vi "UI.vi"(0 "reference in":refnum<class "GUI NV.lvclass">, 5 "error in (no error)":errorcluster) -> (14 "reference out":refnum<class "GUI NV.lvclass">, 19 "error out":errorcluster)   [LabVIEW 2019, in "GUI NV.lvclass"]
uses:
  GUI NV.lvclass
  C:/Users/ANENKOV_V1/Desktop/src/GUI_class/GUI.lvclass
  modbus engine custom/MB_ENGINE_class/Engine Alarms.ctl
  modbus engine custom/MB_ENGINE_class/Settings.ctl
  modbus engine custom/MB_ENGINE_class/cmd enum.ctl
  modbus engine custom/MB_ENGINE_class/Engine State.ctl
  TypeDef/Needle Valve Settings.ctl
  modbus engine custom/MB_ENGINE_class/Limits Status.ctl
  GUI_class/GUI.lvclass/GUI.ctl
  TypeDef/Needle Valve Data.ctl
  TypeDef/Needle Valve State.ctl
  SV_Wrap/SharedVariableWrapper.lvclass/SharedVariableWrapper.ctl
  MessageAMC_class/MessageAMC.lvclass
  C:/Users/ANENKOV_V1/Desktop/src/MessageInterface_class/MessageInterface.lvclass
  1d603503-2144-48e8-a995-f81b8b527575.vi
  8a81be2e-f949-43bf-aca8-28cc7a7f0a37.vi
  d3712f08-a2f0-4b08-adfd-5b0c4b698223.vi
  1b4fed76-272f-4eb9-b435-1b7916789d73.vi
  d0ca9bf2-7cd9-4c29-a03d-de1c10393a74.vi
  0872259c-c1b7-4622-8eff-96544e628326.vi
  9c882fec-a0e6-4663-a7fe-14c8a64433d0.vi
  GUI_class/Set Win State.vi
  GUI_class/protected/GetSheredData.vi
  1b4fed76-272f-4eb9-b435-1b7916789d73.vi/a620cbe0-d7b3-4cdc-ae28-4bc688216dd7.vi
  SV_Wrap/Write Var Info.vi
  SV_Wrap/Read Var Info.vi
  d0ca9bf2-7cd9-4c29-a03d-de1c10393a74.vi/168a1798-03ba-412e-8d8f-3bc5fd34782a.vi
  0872259c-c1b7-4622-8eff-96544e628326.vi/c08680f8-4eaf-4e08-9f5a-be355d832679.vi
  SV_Wrap/Read connection str.vi
  <userlib>/_OpenG.lib/time/time.llb/Tick Count (ms)__ogtk.vi
  GUI_class/GUI.lvclass
  MessageInterface_class/MessageInterface.lvclass
  SV_Wrap/SharedVariableWrapper.lvclass
  modbus engine custom/MB_ENGINE_class/MB_ENGINE.lvclass
panel:
  in  "stop 2":bool
  in  "clear chart":bool
  in  "ziro angl":bool
  out "Limits":T1
  out "Name":string
  in  "Needle Valve Settings":T2={"average size"=0, "open force"=12, "close force"=12, "open settings"={"ACC Steps Per Sec^2"=0, "DEC Steps Per Sec^2"=0, "Min Velosity Step Per Sec"=0, "Max Velosity Step Per Sec"=0, "MicroStep"=0}, "close settings"={"ACC Steps Per Sec^2"=0, "DEC Steps Per Sec^2"=0, "Min Velosity Step Per Sec"=0, "Max Velosity Step Per Sec"=0, "MicroStep"=0}, "Offset angle"=0.0} caption="Settings" {"close force" min=10 max=100; "open force" min=10 max=100; "average size" min=5 max=1000}
  in  "Engine State":T4 items=["ACCELERATING", "DECELERATINGTOSTOP", "DECELERATING", "STEADY", "INDEX_ACCEL", "NDEX_RUN", "INDEX_DECEL", "INDEX_DWELL", "INACTIVE", "STANDBY", "STANDBYTOINACTIVE"]
  out "String 2":string
  out "String":string
  in  "clear fault":bool
  in  "stop":bool
  in  "close":bool
  in  "open":bool
  in  "Set_cmd":bool
  in  "cmd to write":T5 items=["0 Idle"=0, "1 GoTo Absolute Position"=1, "2 GoTo Relative"=2, "10 GoTo Home Position"=10, "11 Set Home Position"=11, "12 Set FindHome Mode"=12, "13 Reset FindHome Mode"=13, "14 Get FindHome State"=14, "20 Hard Stop"=20, "21 HiZ Stop"=21, "22 Soft Stop"=22, "30 Clear Fault"=30, "40 Encoder Set Home"=40, "70 Driver Init"=70]
  out "Kinematic":T3
  out "Waveform Chart - Dark 3":dbl(graph) caption="Угол"
  out "encoder":i32(graph) caption="Энкодер"
  out "step":i32(graph) caption="ШАГ"
  out "Alarms":T6
  out "DO 19":bool
  out "Not Connect":bool caption="Подключение"
  in  "stop":bool
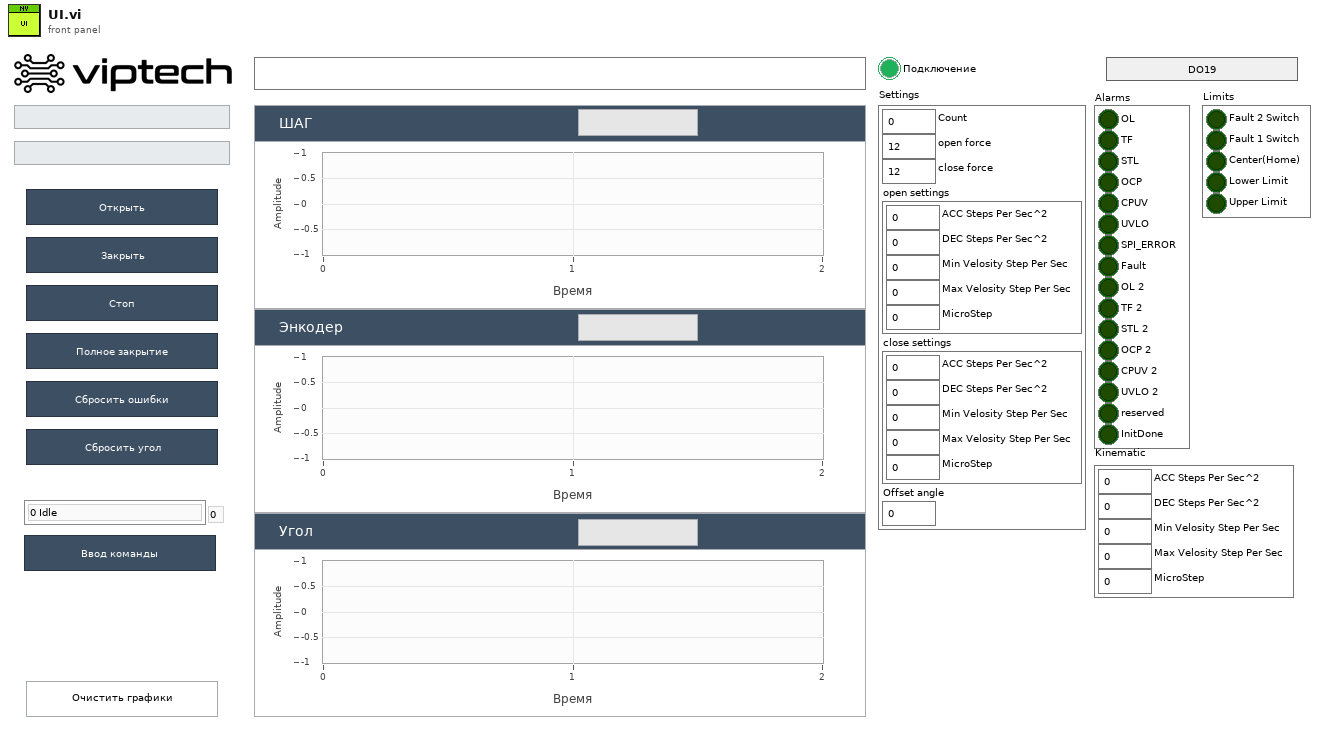
[diagram p1: front panel]
types:
  T1 = typedef "MB_ENGINE.lvclass/Limits Status.ctl" = cluster{"Fault 2 Switch":bool, "Fault 1 Switch":bool, "Center(Home)":bool, "Lower Limit":bool, "Upper Limit":bool}
  T2 = typedef "Needle Valve Settings.ctl" = cluster{"average size":i32, "open force":u16, "close force":u16, "open settings":T3, "close settings":T3, "Offset angle":dbl}
  T3 = typedef "MB_ENGINE.lvclass/Settings.ctl" = cluster{"ACC Steps Per Sec^2":u16, "DEC Steps Per Sec^2":u16, "Min Velosity Step Per Sec":u16, "Max Velosity Step Per Sec":u16, "MicroStep":u16}
  T4 = typedef "MB_ENGINE.lvclass/Engine State.ctl" = u16
  T5 = typedef "MB_ENGINE.lvclass/cmd enum.ctl" = u16
  T6 = typedef "MB_ENGINE.lvclass/Engine Alarms.ctl" = cluster{"OL":bool, "TF":bool, "STL":bool, "OCP":bool, "CPUV":bool, "UVLO":bool, "SPI_ERROR":bool, "Fault":bool, "OL 2":bool, "TF 2":bool, "STL 2":bool, "OCP 2":bool, "CPUV 2":bool, "UVLO 2":bool, "reserved":bool, "InitDone":bool}
  T7 = enum32{"Invalid", "Standard", "Closed", "Hidden", "Minimized", "Maximized"}
  T8 = enum32{"invalid app kind", "Development System", "Run Time System", "Student Edition", "Embedded LabVIEW", "Evaluation", "Custom"}
  T9 = typedef "SharedVariableWrapper.lvclass/Config.ctl" = cluster{"connection str":string, "timeout":dbl, "ip":string}
  T10 = cluster{"Core":cluster{"Current VI Reference":refnum<vi>, "Close Panel on Exit?":bool}, "amc":refnum<class "MessageAMC.lvclass">}
  T11 = cluster{"Current VI Reference":refnum<vi>, "Close Panel on Exit?":bool}
  T12 = typedef "Needle Valve Data.ctl" = cluster{"Engine State":T4, "StateValveModbus":T13, "Alarms":T6, "RAW":i32, "Angele":dbl, "Step":i32, "Encoder":i32, "Kinematic":T3, "Limits":T1, "EncoderMax":i32, "Counter Max Dont Update":i32, "EncoderMin":i32, "Counter Min Dont Update":i32, "Prepere Counter":i32, "STEP INIT":i32, "offset - Angel":dbl}
  T13 = typedef "Needle Valve State.ctl" = enum16{"STOPED", "CLOSED", "OPENED", "OPENING", "CLOSING", "FULL_CLOSE"}
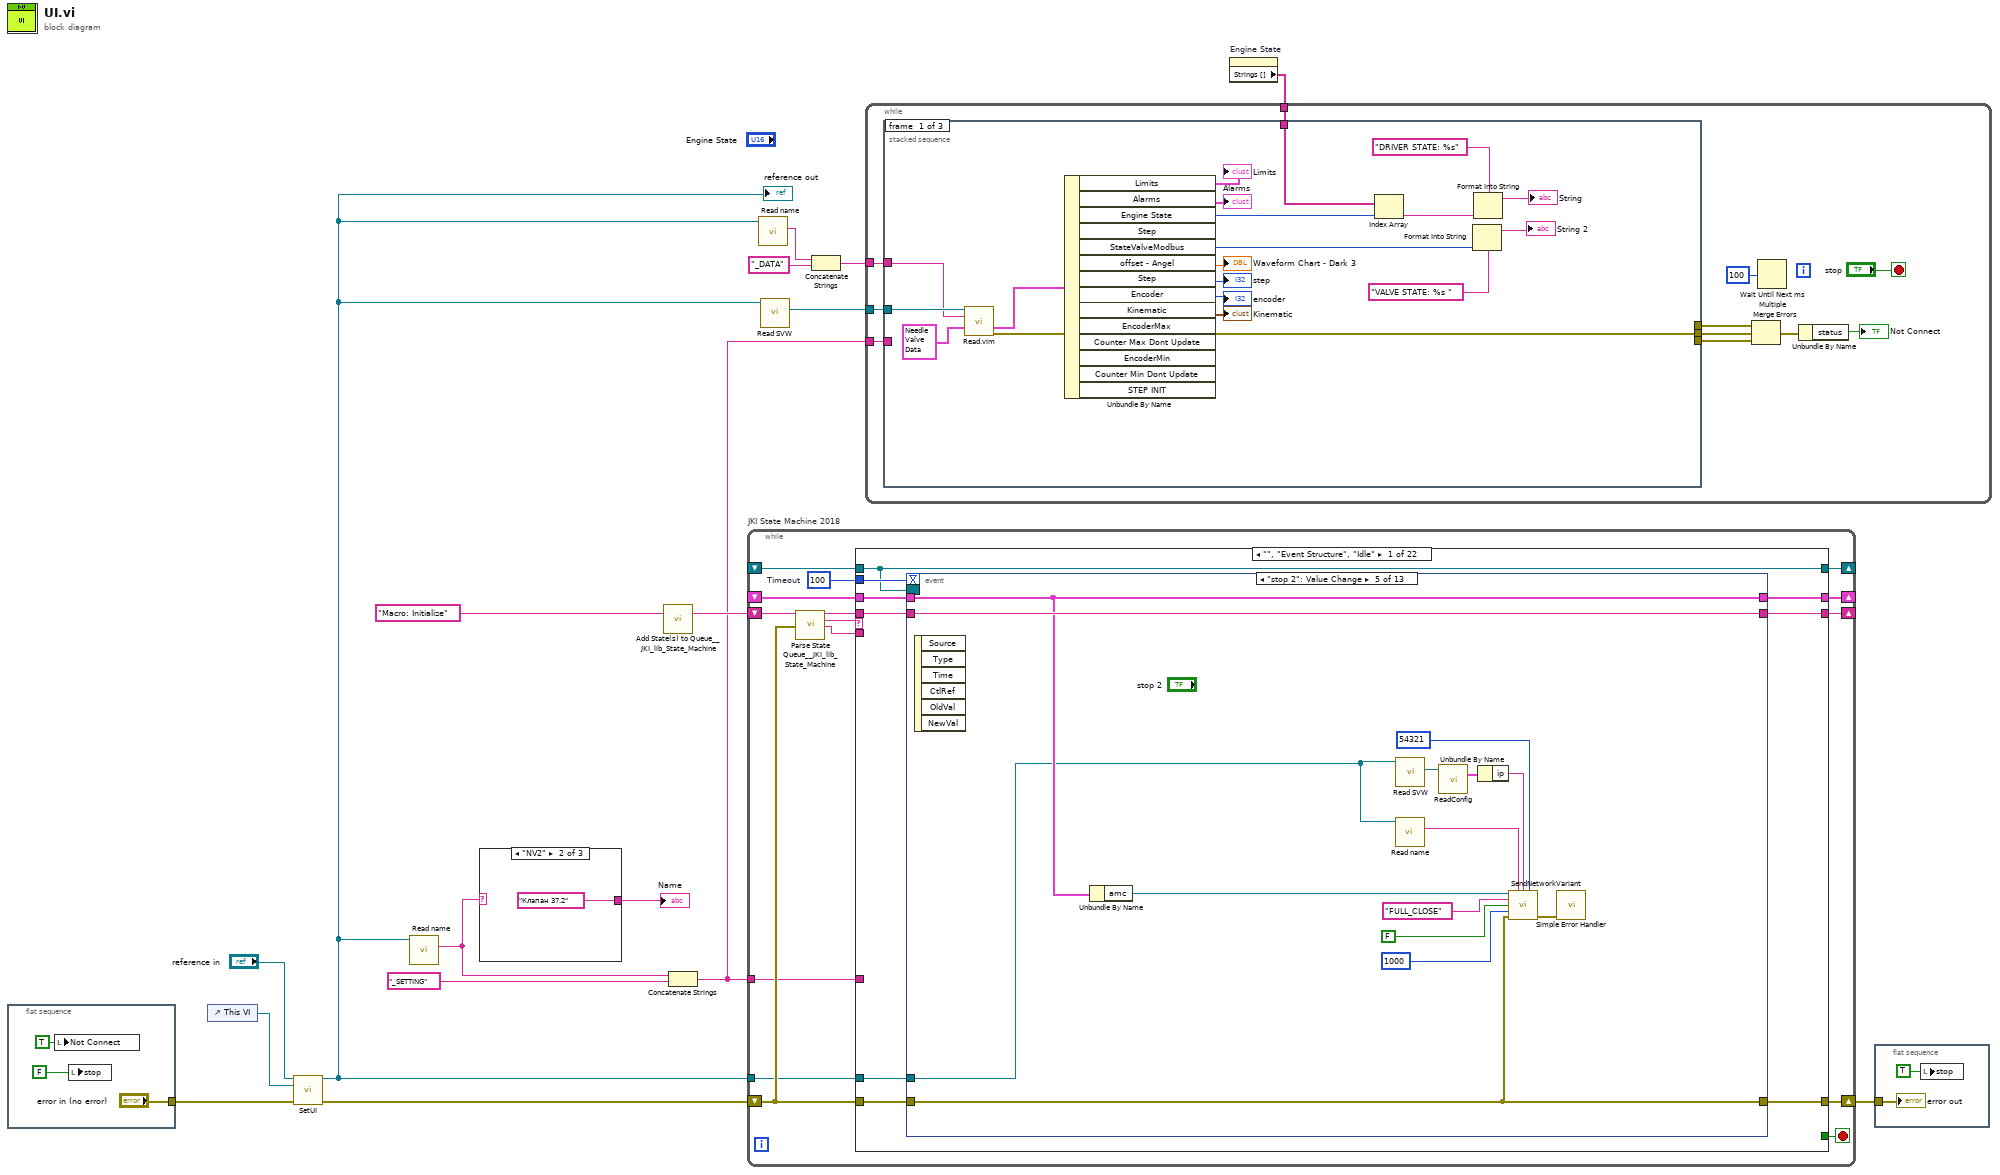
[diagram p0: block diagram]
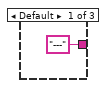
[diagram p2: hidden frame]
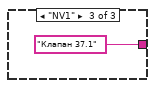
[diagram p3: hidden frame]
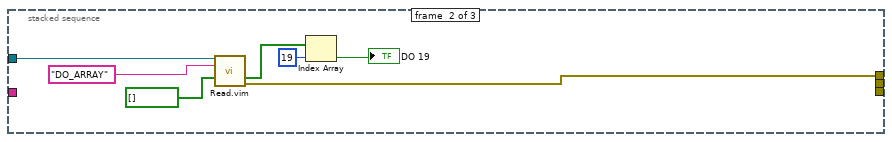
[diagram p4: hidden frame]
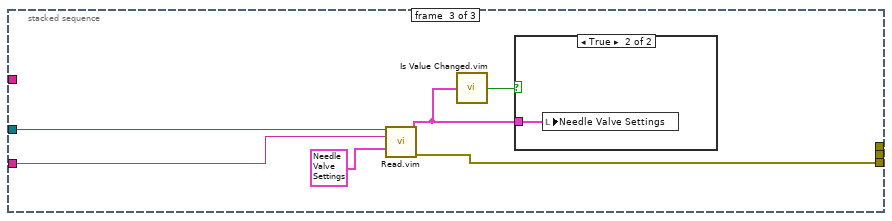
[diagram p5: hidden frame]
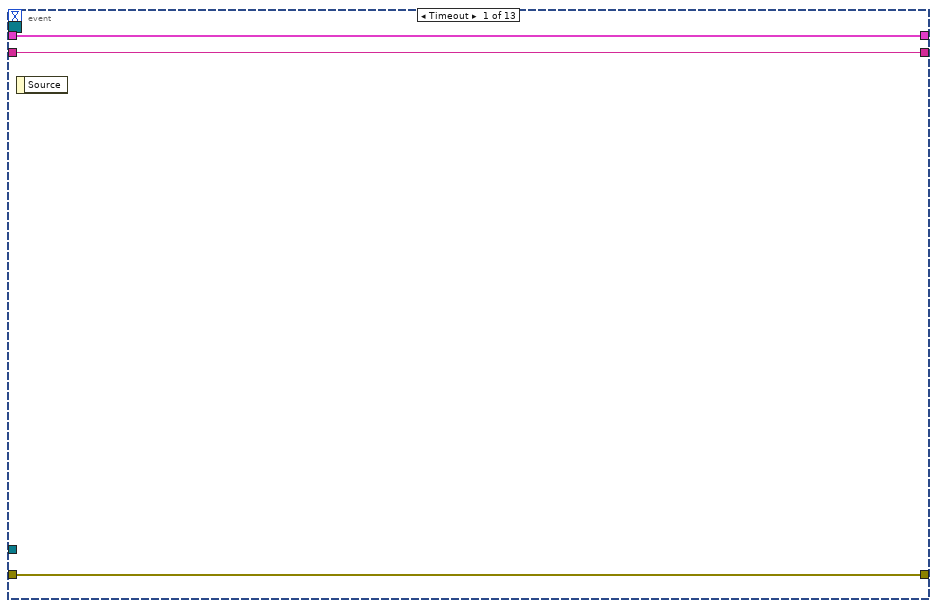
[diagram p7: hidden frame]
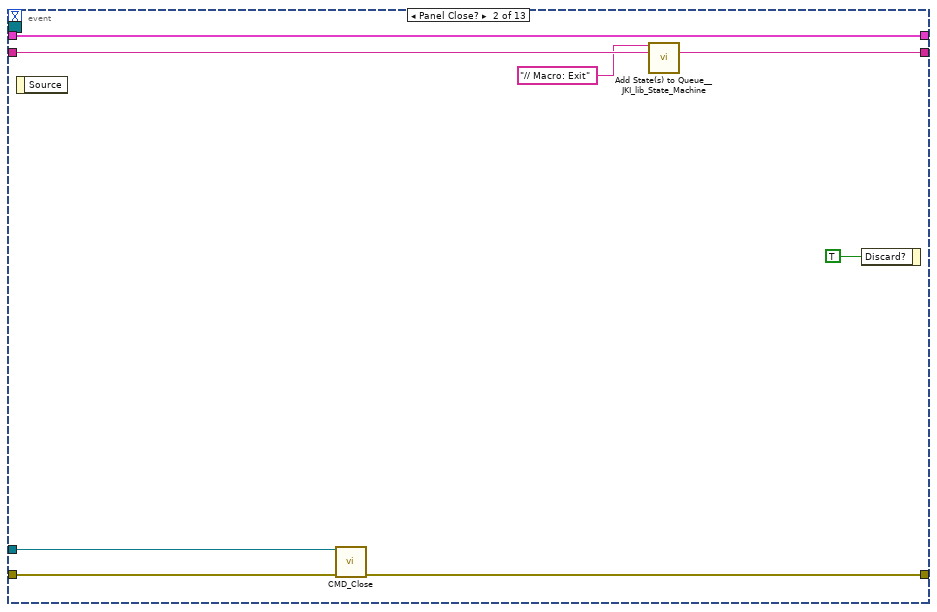
[diagram p8: hidden frame]
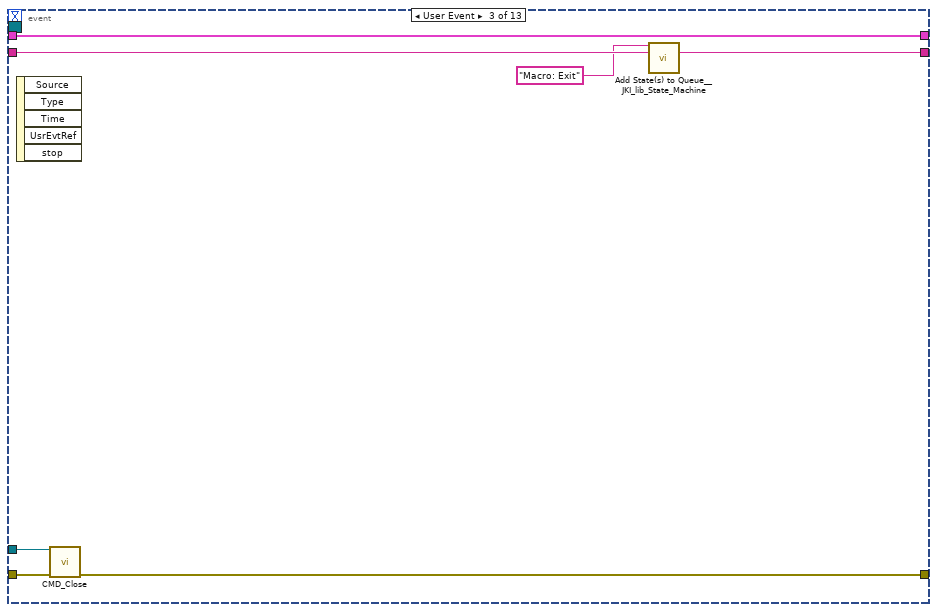
[diagram p9: hidden frame]
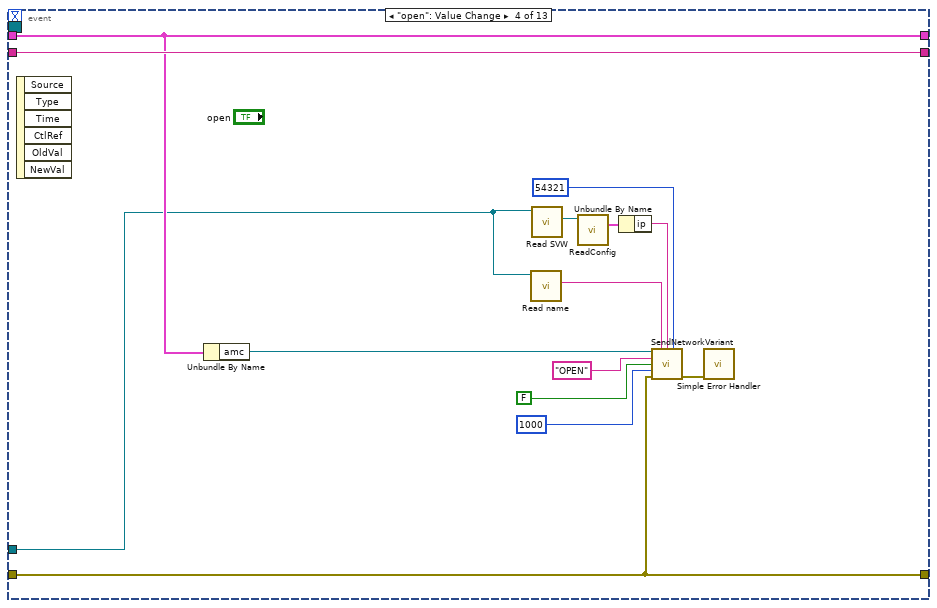
[diagram p10: hidden frame]
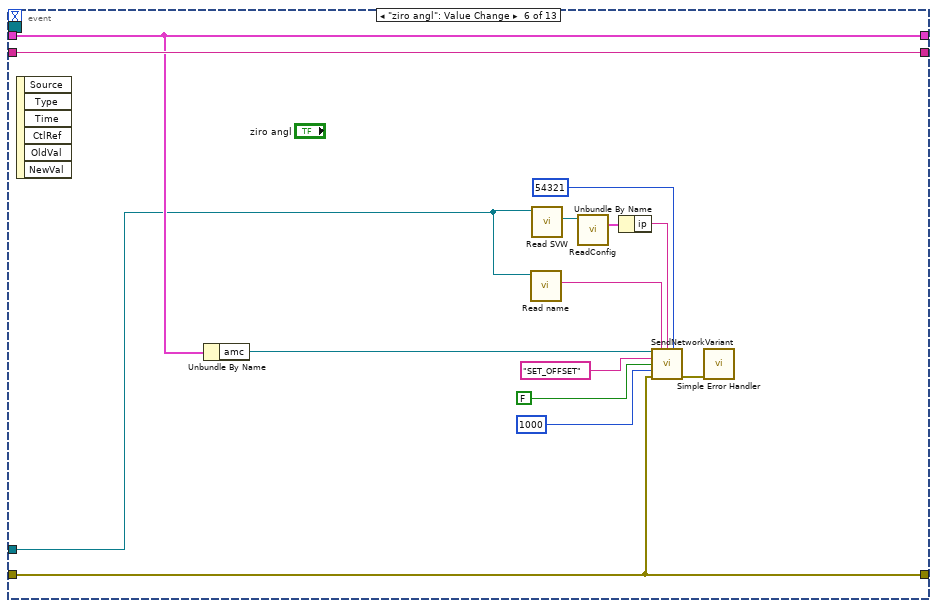
[diagram p11: hidden frame]
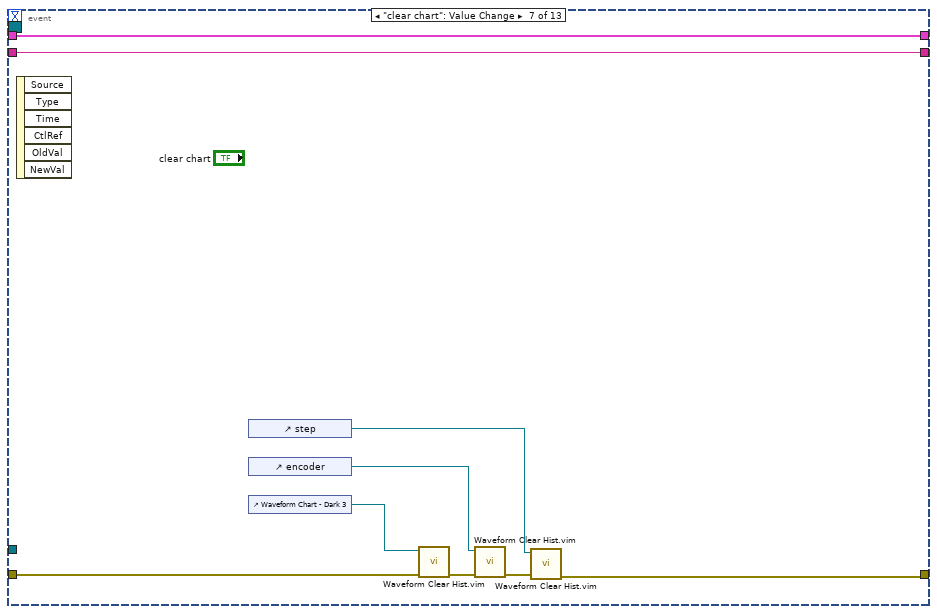
[diagram p12: hidden frame]
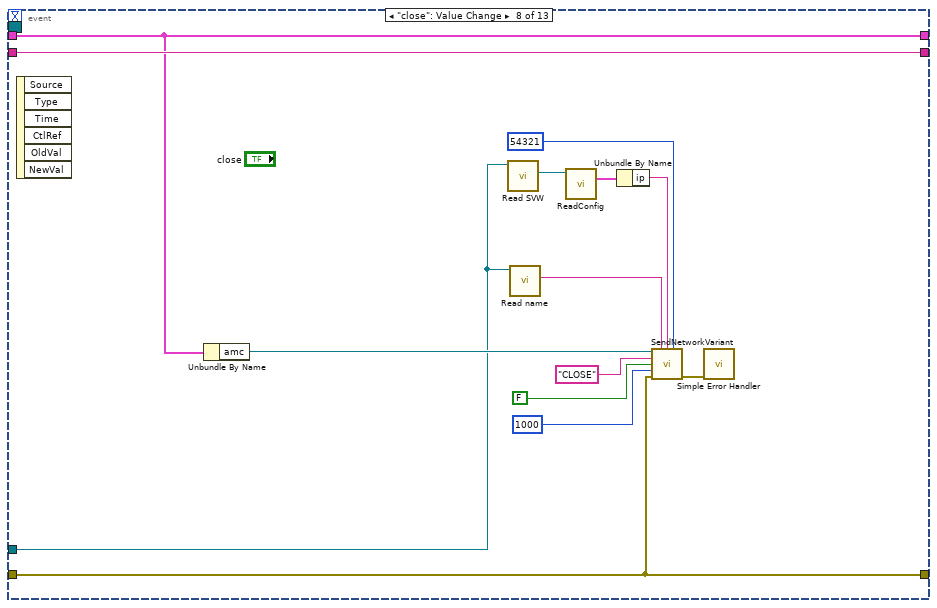
[diagram p13: hidden frame]
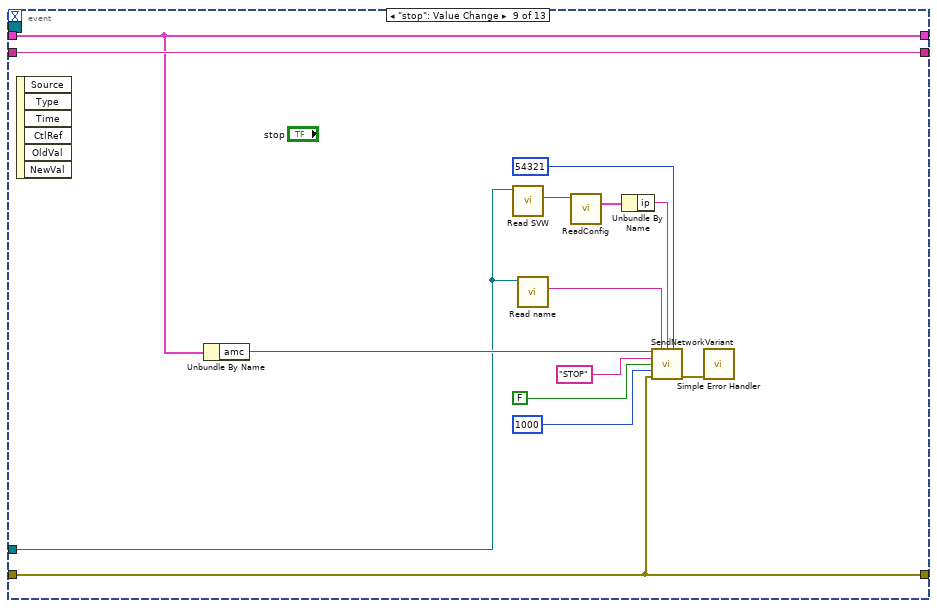
[diagram p14: hidden frame]
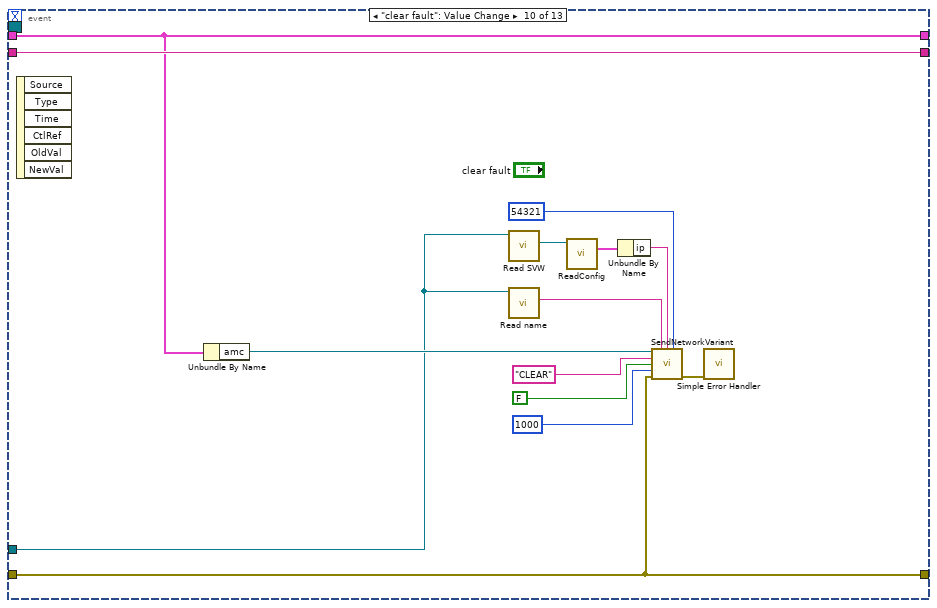
[diagram p15: hidden frame]
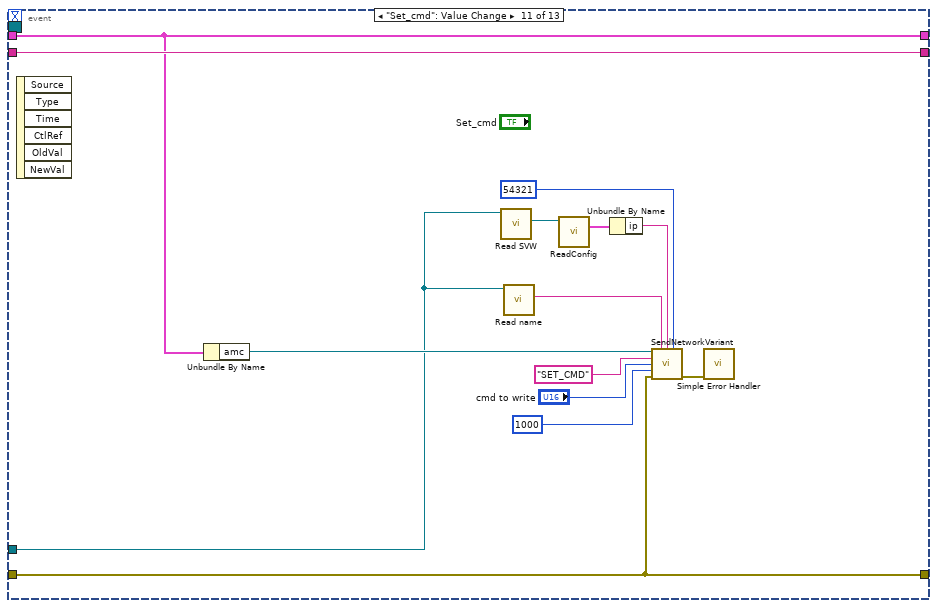
[diagram p16: hidden frame]
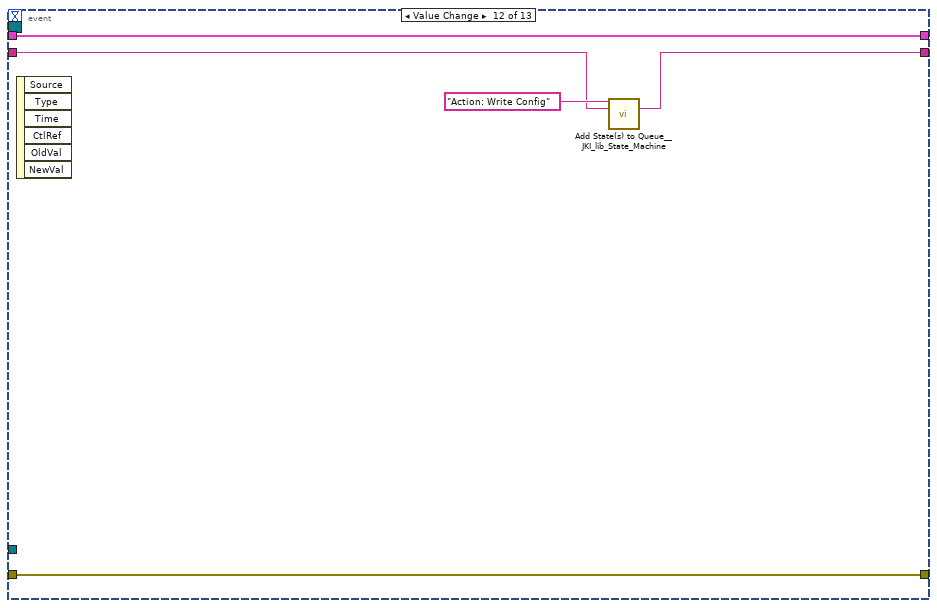
[diagram p17: hidden frame]
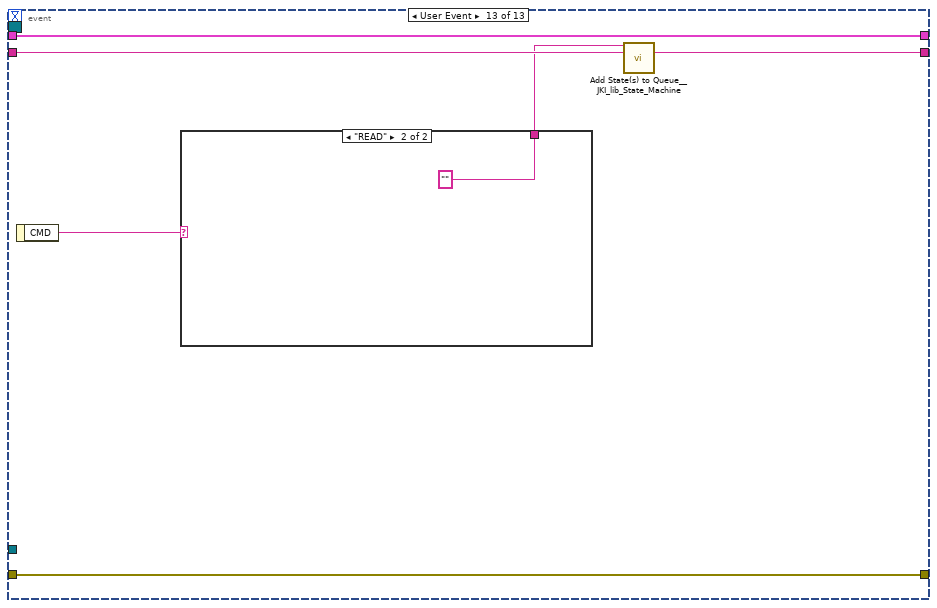
[diagram p18: hidden frame]
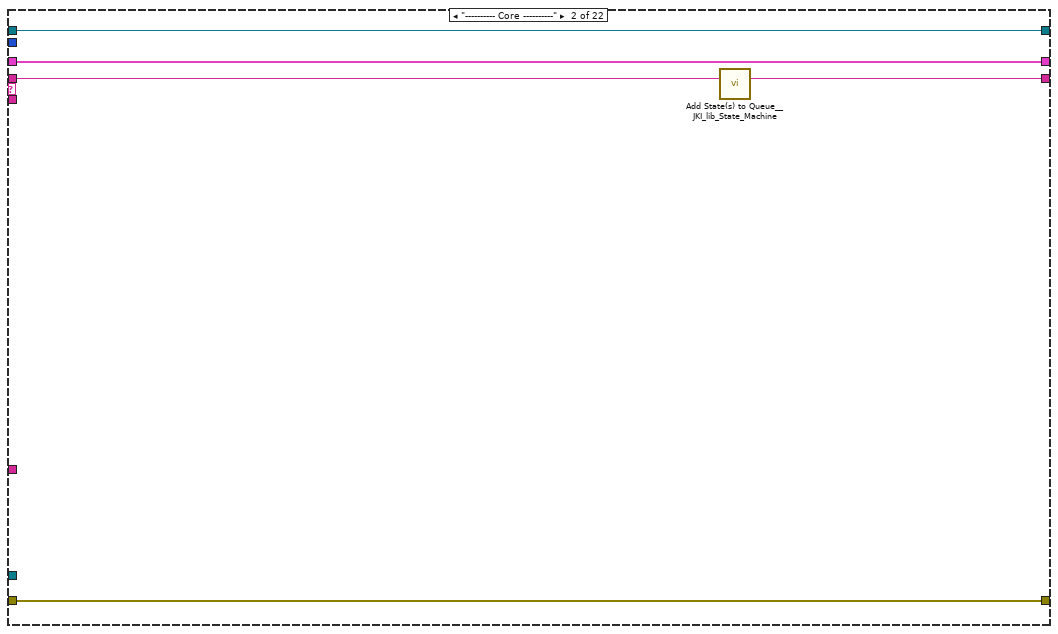
[diagram p20: hidden frame]
diagram:
  n1 = flat-sequence {
    tunnel: ["error in (no error)"] -> w14
    frame #0 {
      n2 = local write "Not Connect"(TRUE ("Connect")) -> ()
      n3 = local write "stop"(FALSE ("stop")) -> ()
    }
  }
  n4 = control-ref of="This VI"() -> (w12:refnum<vi>)
  n5 = call "SetUI.vi"("reference in"="reference in", "UI VI"=w12, "error in (no error)"=w14) -> ("reference out"=w4:refnum<class "GUI NV.lvclass">, "error out"=w11:errorcluster)  [unwired: 11 in]
  "reference out" <- w4
  n6 = call "Read name.vi"("GUI in"=w4) -> ("name"=w2:string)  [unwired: 9 in, 1 out]
  n7 = case shown="\"NV2\"" w2 {
    tunnel: ["---" "Клапан 37.2" "Клапан 37.1"] -> w1
    frame Default {
    }
    frame "NV2" {
    }
    frame "NV1" {
    }
  }
  "Name" <- w1
  n8 = call <vilib>:"Add State(s) to Queue__JKI_lib_State_Machine.vi"("State(s) in (\"\")"="Macro: Initialize") -> ("States Out"=w17:string)  [unwired: 14 in]
  n9 = Concatenate Strings(w2, "_SETTING" ("name")) -> (w3:string)
  n10 = while "JKI State Machine 2018" {
    shift-right: [w31] -> _
    shift-left: _ -> [w30]
    shift-right: [w34] -> w15
    shift-left: w11 -> [w28]
    shift-right: [w33] -> _
    shift-left: w17 -> [w35]
    tunnel: w4 -> [w27]
    shift-right: [w26] -> _
    shift-left: _ -> [w25]
    tunnel: w3 -> [w24]
    stop <- w32 stop-if-true
    w29 = 100  # Timeout
    n11 = call <vilib>:"Parse State Queue__JKI_lib_State_Machine.vi"("State Queue"=w35, "Error In (no error)"=w28) -> ("Remaining States"=w37:string, "Current State"=w38:string, "Arguments"=w36:string)  [unwired: 11 in]
    n12 = case shown="\"\", \"Event Structure\", \"Idle\"" w38 {
      selector: w38 -> [_ _ w191 _ _ _ _ _ _ _ _ _ _ _ _ _ _ _ _ _ _ _]
      tunnel: w37 -> [w47 w189 w195 w215 w222 w230 w235 w244 w251 w256 w264 w270 w275 w279 w286 w298 w368 w374 w380 w392 w396 w403]
      tunnel: w36 -> [_ _ _ _ _ _ _ _ _ _ _ _ _ _ w281 w292 _ _ _ _ _ _]
      tunnel: w30 -> [w45 w186 w193 w208 w219 w225 w232 _ w246 w253 w263 w268 w272 w278 w284 w294 w365 w371 w377 w389 w394 w398]
      tunnel: [w44 w187 w197 w212 errorcluster {"status"=FALSE, "code"=0, "source"=""} ("error out") w228 w233 w237 w247 w254 w261 w265 w273 w277 w282 w295 w366 w372 w378 w390 w395 w400] -> w34
      tunnel: w28 -> [w43 w187 w196 w212 w218 w228 w233 w238 w248 w254 w260 w266 w273 w277 w283 w296 w366 w372 w378 w390 w395 w401]
      tunnel: [w46 w188 w194 w214 w221 w229 w234 w244 w250 w255 w264 w269 w274 w279 w285 w297 w367 w373 w379 w391 w396 w403] -> w33
      tunnel: [_ _ _ _ _ TRUE _ _ _ _ _ _ _ _ _ _ _ _ _ _ _ _] -> w32
      tunnel: [w42 w186 w193 w213 w219 w225 w232 w243 w246 w253 w263 w268 w272 w278 w284 w294 w365 w371 w377 w389 w394 w398] -> w31
      tunnel: w29 -> [w41 _ _ _ _ _ _ _ _ _ _ _ _ _ _ _ _ _ _ _ _ _]
      tunnel: w27 -> [w40 _ _ _ _ _ _ _ _ _ w259 _ _ _ _ _ _ _ _ _ _ w399]
      tunnel: [w39 w185 w190 w202 w216 w226 w231 w241 w245 w252 w262 w267 w271 w276 w280 w291 w364 w369 w375 w382 w393 w402] -> w26
      tunnel: w25 -> [w39 w185 w190 w202 w216 w226 w231 w241 w245 w252 _ w267 w271 w276 w280 w291 w364 w369 w375 w382 w393 w402]
      tunnel: w24 -> [_ _ _ _ _ _ _ _ _ _ _ _ _ _ _ _ _ _ _ _ _ _]
      frame "", "Event Structure", "Idle" {
        n13 = event shown="[4] \"stop 2\": Value Change" {
          selector: w39 -> [_ _ _ _ _ _ _ _ _ _ _ _ _]
          dyn-events: _ -> [_ _ _ _ _ _ _ _ _ _ _ _ _]
          timeout: w41 -> [_ _ _ _ _ _ _ _ _ _ _ _ _]
          tunnel: w47 -> [w50 w58 w65 w79 w93 w107 w116 w130 w144 w158 w172 w174 w180]
          tunnel: [w50 w57 w64 w79 w93 w107 w116 w130 w144 w158 w172 w173 w181] -> w46
          tunnel: w45 -> [w48 w56 w63 w73 w87 w101 w115 w124 w138 w152 w166 w176 w182]
          tunnel: [w49 w51 w59 w68 w82 w96 w111 w119 w133 w147 w162 w177 w183] -> w44
          tunnel: w43 -> [w49 w52 w60 w68 w82 w96 w114 w119 w133 w147 w162 w177 w183]
          tunnel: [w48 w56 w63 w73 w87 w101 w115 w124 w138 w152 w166 w176 w182] -> w42
          tunnel: w40 -> [_ w53 w61 w66 w80 w94 _ w118 w132 w146 w160 _ _]
          event Timeout {
            n14 = event-data() -> ()  [unwired: 1 in, 1 out]
          }
          event Panel Close? {
            n15 = event-data() -> ()  [unwired: 1 in, 1 out]
            n16 = call "CMD_Close.vi"("reference in"=w53, "error in (no error)"=w52) -> ("error out"=w51:errorcluster)  [unwired: 12 in, 1 out]
            n17 = call <vilib>:"Add State(s) to Queue__JKI_lib_State_Machine.vi"("State(s) in Front (\"\")"="// Macro: Exit", "State(s) in (\"\")"=w58) -> ("States Out"=w57:string)  [unwired: 13 in]
            n18 = event-data("Discard?"=TRUE) -> ()  [unwired: 1 in, 1 out]
          }
          event User Event {
            n19 = event-data() -> ()  [unwired: 1 in, 5 out]
            n20 = call "CMD_Close.vi"("reference in"=w61, "error in (no error)"=w60) -> ("error out"=w59:errorcluster)  [unwired: 12 in, 1 out]
            n21 = call <vilib>:"Add State(s) to Queue__JKI_lib_State_Machine.vi"("State(s) in Front (\"\")"="Macro: Exit", "State(s) in (\"\")"=w65) -> ("States Out"=w64:string)  [unwired: 13 in]
          }
          event "open": Value Change {
            n22 = event-data() -> ()  [unwired: 1 in, 6 out]
            n23 = Unbundle By Name(w73) -> ("amc"=w72:refnum<class "MessageAMC.lvclass">)
            n24 = call "Read name.vi"("GUI in"=w66) -> ("name"=w67:string)  [unwired: 9 in, 1 out]
            n25 = call "Read SVW.vi"("GUI in"=w66) -> ("SharedVariableWrapper.lvclass"=w75:refnum<class "SharedVariableWrapper.lvclass">)  [unwired: 10 in]
            n26 = call "ReadConfig.vi"("SharedVariableWrapper in"=w75) -> ("config"=w74:T9)  [unwired: 12 in, 2 out]
            n27 = Unbundle By Name(w74) -> ("ip"=w71:string)
            n28 = call "SendNetworkVariant.vi"("reference in"=w72, "receiver process"=w67, "receiver host"=w71, "receiver port (0)"=u16 54321, "name"="OPEN", "data"=FALSE, "timeout (25000 ms)"=1000, "error in (no error)"=w68) -> ("error out"=w69:errorcluster)  [unwired: 5 in, 2 out]
            n29 = call <vilib>:"Simple Error Handler.vi"("error in (no error)"=w69) -> ()  [unwired: 4 in, 5 out]
          }
          event "stop 2": Value Change {
            n30 = event-data() -> ()  [unwired: 1 in, 6 out]
            n31 = Unbundle By Name(w87) -> ("amc"=w86:refnum<class "MessageAMC.lvclass">)
            n32 = call "Read name.vi"("GUI in"=w80) -> ("name"=w81:string)  [unwired: 9 in, 1 out]
            n33 = call "Read SVW.vi"("GUI in"=w80) -> ("SharedVariableWrapper.lvclass"=w89:refnum<class "SharedVariableWrapper.lvclass">)  [unwired: 10 in]
            n34 = call "ReadConfig.vi"("SharedVariableWrapper in"=w89) -> ("config"=w88:T9)  [unwired: 12 in, 2 out]
            n35 = Unbundle By Name(w88) -> ("ip"=w85:string)
            n36 = call "SendNetworkVariant.vi"("reference in"=w86, "receiver process"=w81, "receiver host"=w85, "receiver port (0)"=u16 54321, "name"="FULL_CLOSE", "data"=FALSE, "timeout (25000 ms)"=1000, "error in (no error)"=w82) -> ("error out"=w83:errorcluster)  [unwired: 5 in, 2 out]
            n37 = call <vilib>:"Simple Error Handler.vi"("error in (no error)"=w83) -> ()  [unwired: 4 in, 5 out]
          }
          event "ziro angl": Value Change {
            n38 = event-data() -> ()  [unwired: 1 in, 6 out]
            n39 = Unbundle By Name(w101) -> ("amc"=w100:refnum<class "MessageAMC.lvclass">)
            n40 = call "Read name.vi"("GUI in"=w94) -> ("name"=w95:string)  [unwired: 9 in, 1 out]
            n41 = call "Read SVW.vi"("GUI in"=w94) -> ("SharedVariableWrapper.lvclass"=w103:refnum<class "SharedVariableWrapper.lvclass">)  [unwired: 10 in]
            n42 = call "ReadConfig.vi"("SharedVariableWrapper in"=w103) -> ("config"=w102:T9)  [unwired: 12 in, 2 out]
            n43 = Unbundle By Name(w102) -> ("ip"=w99:string)
            n44 = call "SendNetworkVariant.vi"("reference in"=w100, "receiver process"=w95, "receiver host"=w99, "receiver port (0)"=u16 54321, "name"="SET_OFFSET", "data"=FALSE, "timeout (25000 ms)"=1000, "error in (no error)"=w96) -> ("error out"=w97:errorcluster)  [unwired: 5 in, 2 out]
            n45 = call <vilib>:"Simple Error Handler.vi"("error in (no error)"=w97) -> ()  [unwired: 4 in, 5 out]
          }
          event "clear chart": Value Change {
            n46 = event-data() -> ()  [unwired: 1 in, 6 out]
            n47 = control-ref of="step"() -> (w108:refnum<vi>)
            n48 = control-ref of="encoder"() -> (w109:refnum<vi>)
            n49 = control-ref of="Waveform Chart - Dark 3"() -> (w110:refnum<vi>)
            n50 = call "Waveform Clear Hist.vim"("error in (no error)"=w114, "WaveformChart in"=w110) -> ("error out"=w113:errorcluster)  [unwired: 9 in]
            n51 = call "Waveform Clear Hist.vim"("error in (no error)"=w113, "WaveformChart in"=w109) -> ("error out"=w112:errorcluster)  [unwired: 9 in]
            n52 = call "Waveform Clear Hist.vim"("error in (no error)"=w112, "WaveformChart in"=w108) -> ("error out"=w111:errorcluster)  [unwired: 9 in]
          }
          event "close": Value Change {
            n53 = event-data() -> ()  [unwired: 1 in, 6 out]
            n54 = Unbundle By Name(w124) -> ("amc"=w123:refnum<class "MessageAMC.lvclass">)
            n55 = call "Read SVW.vi"("GUI in"=w118) -> ("SharedVariableWrapper.lvclass"=w126:refnum<class "SharedVariableWrapper.lvclass">)  [unwired: 10 in]
            n56 = call "Read name.vi"("GUI in"=w118) -> ("name"=w117:string)  [unwired: 9 in, 1 out]
            n57 = call "ReadConfig.vi"("SharedVariableWrapper in"=w126) -> ("config"=w125:T9)  [unwired: 12 in, 2 out]
            n58 = Unbundle By Name(w125) -> ("ip"=w122:string)
            n59 = call "SendNetworkVariant.vi"("reference in"=w123, "receiver process"=w117, "receiver host"=w122, "receiver port (0)"=u16 54321, "name"="CLOSE", "data"=FALSE, "timeout (25000 ms)"=1000, "error in (no error)"=w119) -> ("error out"=w120:errorcluster)  [unwired: 5 in, 2 out]
            n60 = call <vilib>:"Simple Error Handler.vi"("error in (no error)"=w120) -> ()  [unwired: 4 in, 5 out]
          }
          event "stop": Value Change {
            n61 = event-data() -> ()  [unwired: 1 in, 6 out]
            n62 = Unbundle By Name(w138) -> ("amc"=w137:refnum<class "MessageAMC.lvclass">)
            n63 = call "Read SVW.vi"("GUI in"=w132) -> ("SharedVariableWrapper.lvclass"=w140:refnum<class "SharedVariableWrapper.lvclass">)  [unwired: 10 in]
            n64 = call "Read name.vi"("GUI in"=w132) -> ("name"=w131:string)  [unwired: 9 in, 1 out]
            n65 = call "ReadConfig.vi"("SharedVariableWrapper in"=w140) -> ("config"=w139:T9)  [unwired: 12 in, 2 out]
            n66 = Unbundle By Name(w139) -> ("ip"=w136:string)
            n67 = call "SendNetworkVariant.vi"("reference in"=w137, "receiver process"=w131, "receiver host"=w136, "receiver port (0)"=u16 54321, "name"="STOP", "data"=FALSE, "timeout (25000 ms)"=1000, "error in (no error)"=w133) -> ("error out"=w134:errorcluster)  [unwired: 5 in, 2 out]
            n68 = call <vilib>:"Simple Error Handler.vi"("error in (no error)"=w134) -> ()  [unwired: 4 in, 5 out]
          }
          event "clear fault": Value Change {
            n69 = event-data() -> ()  [unwired: 1 in, 6 out]
            n70 = Unbundle By Name(w152) -> ("amc"=w151:refnum<class "MessageAMC.lvclass">)
            n71 = call "Read SVW.vi"("GUI in"=w146) -> ("SharedVariableWrapper.lvclass"=w154:refnum<class "SharedVariableWrapper.lvclass">)  [unwired: 10 in]
            n72 = call "Read name.vi"("GUI in"=w146) -> ("name"=w145:string)  [unwired: 9 in, 1 out]
            n73 = call "ReadConfig.vi"("SharedVariableWrapper in"=w154) -> ("config"=w153:T9)  [unwired: 12 in, 2 out]
            n74 = Unbundle By Name(w153) -> ("ip"=w150:string)
            n75 = call "SendNetworkVariant.vi"("reference in"=w151, "receiver process"=w145, "receiver host"=w150, "receiver port (0)"=u16 54321, "name"="CLEAR", "data"=FALSE, "timeout (25000 ms)"=1000, "error in (no error)"=w147) -> ("error out"=w148:errorcluster)  [unwired: 5 in, 2 out]
            n76 = call <vilib>:"Simple Error Handler.vi"("error in (no error)"=w148) -> ()  [unwired: 4 in, 5 out]
          }
          event "Set_cmd": Value Change {
            n77 = event-data() -> ()  [unwired: 1 in, 6 out]
            n78 = Unbundle By Name(w166) -> ("amc"=w165:refnum<class "MessageAMC.lvclass">)
            n79 = call "Read SVW.vi"("GUI in"=w160) -> ("SharedVariableWrapper.lvclass"=w168:refnum<class "SharedVariableWrapper.lvclass">)  [unwired: 10 in]
            n80 = call "Read name.vi"("GUI in"=w160) -> ("name"=w159:string)  [unwired: 9 in, 1 out]
            n81 = call "ReadConfig.vi"("SharedVariableWrapper in"=w168) -> ("config"=w167:T9)  [unwired: 12 in, 2 out]
            n82 = Unbundle By Name(w167) -> ("ip"=w164:string)
            n83 = call "SendNetworkVariant.vi"("reference in"=w165, "receiver process"=w159, "receiver host"=w164, "receiver port (0)"=u16 54321, "name"="SET_CMD", "data"="cmd to write", "timeout (25000 ms)"=1000, "error in (no error)"=w162) -> ("error out"=w163:errorcluster)  [unwired: 5 in, 2 out]
            n84 = call <vilib>:"Simple Error Handler.vi"("error in (no error)"=w163) -> ()  [unwired: 4 in, 5 out]
          }
          event Value Change {
            n85 = event-data() -> ()  [unwired: 1 in, 6 out]
            n86 = call <vilib>:"Add State(s) to Queue__JKI_lib_State_Machine.vi"("State(s) in Front (\"\")"="Action: Write Config" ("State(s) in Front (\"\")"), "State(s) in (\"\")"=w174) -> ("States Out"=w173:string)  [unwired: 13 in]
          }
          event User Event {
            n87 = event-data() -> ("CMD"=w179:string)  [unwired: 1 in]
            n88 = case shown="\"READ\"" w179 {
              tunnel: [_ "" ("State(s) in Front (\"\")")] -> w178
              frame "False", Default {
              }
              frame "READ" {
              }
            }
            n89 = call <vilib>:"Add State(s) to Queue__JKI_lib_State_Machine.vi"("State(s) in Front (\"\")"=w178, "State(s) in (\"\")"=w180) -> ("States Out"=w181:string)  [unwired: 13 in]
          }
        }
      }
      frame "---------- Core ----------" {
        n90 = call <vilib>:"Add State(s) to Queue__JKI_lib_State_Machine.vi"("State(s) in (\"\")"=w189) -> ("States Out"=w188:string)  [unwired: 14 in]
      }
      frame Default {
        w200 = 42 items=["No error", "Argument error", "Memory is full", "Out of zone", "End of file", "File already open", "Generic file I/O error", "File not found", "File permission error", "Disk is full", "Duplicate path", "Too many files open", "System feature not enabled", "Resource file not found", "Cannot add resource", "Resource not found", "Image not found", "Image memory error", "Pen does not exist", "Config type invalid", "Config token not found", "Config parse error", "Config memory error", "Bad external code format", "Bad external code offset", "External code not present", "Null window", "Destroy window error", "Null menu", "Print aborted", "Bad print record", "Print driver error", "Windows error during printing", "Memory error during printing", "Print dialog error", "Generic print error", "Invalid device refnum", "Device not found", "Device parameter error", "Device unit error", "Cannot open device", "Device call aborted", "Generic error", "Cancelled by user", "Object ID too low", "Object ID too high", "Object not in heap", "Unknown heap", "Unknown object (invalid DefProc)", "Unknown object (DefProc not in table)", "Message out of range", "Invalid (null) method", "Unknown message", "Manager call not supported", "Bad address", "Network operation in progress", "Network operation timed out", "Connection is busy", "Network attribute not supported", "Network error", "Address in use", "System out of memory", "Connection aborted", "Connection refused", "Not connected", "Already connected", "Connection closed", "Initialization error (interapplication manager)", "Bad occurrence", "Wait on unbound occurrence handler", "Occurrence queue overflow", "Datalog type conflict", "Unused", "Unrecognized type (interapplication manager)", "Memory corrupt", "Failed to make temporary DLL", "Old CIN version", "Drag socket not found", "Failed to load drop-object", "Failed to register OLE object", "Failed to release OLE object", "Format specifier type mismatch", "Unknown format specifier", "Too few format specifiers", "Too many format specifiers", "Scan failed", "Newer CIN version", "Error converting to variant", "Runtime menu error", "Password tampered", "Variant attribute not found", "Incompatible variant data type", "Event data is not available", "Event Store is not present", "Occurrence is not found", "Event Queue is not created", "Event info is not available", "Refnum passed is NULL", "Error retrieving Class GUID", "Error retrieving CoClass GUID", "Error retrieving TypeLib GUID.", "Bad built application magic bytes.", "Specific driver is different from the specific driver associated with the Logical Name.", "There is no session opened to the class driver.", "Max Error", "MAX - Error with config objects", "MAX - Error loading configuration", "MAX - Group not supported"]
        # "Current State"
        # "Do not delete, rename, or modify this frame.\n(this is used to capture unhandled states and typos)"
        # "Handle mistyped state name (developer tool)"
        n91 = Format Into String(format string="Software Exception: Unhandled State \"%s\"." ("message"), error in=w196, w191) -> (resulting string=w199:string, error out=w198:errorcluster)  [unwired: 1 in]
        n92 = call <vilib>:"Error Cluster From Error Code.vi"("show call chain? (False)"=TRUE, "error in (no error)"=w198, "error message (\"\")"=w199, "error code (0)"=w200) -> ("error out"=w197:errorcluster)  [unwired: 5 in]
        n93 = call <vilib>:"Add State(s) to Queue__JKI_lib_State_Machine.vi"("State(s) in (\"\")"=w195) -> ("States Out"=w194:string)  [unwired: 14 in]
      }
      frame "Initialize Core Data" {
        # "Do not delete, rename, or modify this frame.\n(this is used to determine panel behavior on exit)"
        # "originally closed?"
        # "exe?"
        # "If panel starts closed or is an EXE, then close it when we exit"
        n94 = property class="VI"() -> ("FP.State"=w205:T7)  [unwired: 2 in, 2 out]
        n95 = property class="App"() -> ("App.Kind"=w211:T8)  [unwired: 2 in, 2 out]
        n96 = control-ref of="Current VI Reference"() -> (w206:refnum<vi>)
        n97 = Equal?(x=w205, y=T7."Closed" ("Front Panel Window:State")) -> (x = y?=w203:bool)
        n98 = Equal?(x=w211, y=T8."Run Time System" ("Application:Kind")) -> (x = y?=w209:bool)
        n99 = Or(x=w203, y=w209) -> (x .or. y?=w207:bool)
        n100 = Bundle By Name(cluster=w208, "Core.Current VI Reference"=w206, "Core.Close Panel on Exit?"=w207) -> (w213:T10)
        n101 = call <vilib>:"Add State(s) to Queue__JKI_lib_State_Machine.vi"("State(s) in (\"\")"=w215) -> ("States Out"=w214:string)  [unwired: 14 in]
      }
      frame "Error Handler" {
        # "Unhandled Error -- Display it"
        # "Handle any errors here.\nYou can also output any states to clean-up after errors occur"
        # "Clear error"
        n102 = call <vilib>:"General Error Handler.vi"("error in (no error)"=w218) -> ()  [unwired: 10 in, 5 out]
        n103 = call <vilib>:"Add State(s) to Queue__JKI_lib_State_Machine.vi"("State(s) in Front (\"\")"="/* Post Error States", "State(s) in (\"\")"=w222) -> ("States Out"=w221:string)  [unwired: 13 in]
      }
      frame "Exit" {
        n104 = Unbundle By Name(w225) -> ("amc"=w224:refnum<class "MessageAMC.lvclass">)
        n105 = call-dynamic "Destroy.vi"("reference in"=w224) -> ("error out"=w223:errorcluster)  [unwired: 17 in, 1 out]
        n106 = call <vilib>:"Clear Errors.vi"("error in (no error)"=w223) -> ()  [unwired: 5 in, 2 out]
        n107 = call <vilib>:"Add State(s) to Queue__JKI_lib_State_Machine.vi"("State(s) in (\"\")"=w230) -> ("States Out"=w229:string)  [unwired: 14 in]
      }
      frame "---------- Data ----------" {
        # "Do not put any code in this frame.\n(It is a separator no-op. You can make a copy of this frame to create a new Data frame)"
        n108 = call <vilib>:"Add State(s) to Queue__JKI_lib_State_Machine.vi"("State(s) in (\"\")"=w235) -> ("States Out"=w234:string)  [unwired: 14 in]
      }
      frame "Data: Initialize" {
        w242 = T11 {"Current VI Reference"=refnum, "Close Panel on Exit?"=FALSE}  # Core
        n109 = call "MessageAMC_Create.vi"("reference in"=refnum<class "MessageAMC.lvclass"> refnum, "error in (no error)"=w238, "message queue name"="GUI_NVM_1") -> ("amc"=w239:refnum<class "MessageAMC.lvclass">, "error out"=w237:errorcluster)  [unwired: 15 in]
        n110 = Bundle("Core"=w242, "amc"=w239) -> (w243:T10)  [unwired: 1 in]
      }
      frame "Data: Cleanup" {
        # "Cleanup any data and references, here.\n(this is called automatically, by the Macro: Exit)"
        n111 = Unbundle By Name(w246) -> ("Core.Current VI Reference"=w249:refnum<vi>)
        n112 = Close Reference(reference=w249, error in (no error)=w248) -> (error out=w247:errorcluster)
        n113 = call <vilib>:"Add State(s) to Queue__JKI_lib_State_Machine.vi"("State(s) in (\"\")"=w251) -> ("States Out"=w250:string)  [unwired: 14 in]
      }
      frame "---------- Events ----------" {
        # "Do not put any code in this frame.\n(It is a separator no-op. You can make a copy of this frame to create a new UI frame)"
        n114 = call <vilib>:"Add State(s) to Queue__JKI_lib_State_Machine.vi"("State(s) in (\"\")"=w256) -> ("States Out"=w255:string)  [unwired: 14 in]
      }
      frame "Events: Register" {
        n115 = call "Read stop event.vi"("GUI in"=w259) -> ("cmd event"=w257:refnum<user-event>, "stop event"=w258:refnum<user-event>)  [unwired: 8 in, 1 out]
        n116 = register-events(error in=w260, w258, w257) -> (reference out=w262:refnum<event-registration>, error out=w261:errorcluster)  [unwired: 1 in]
      }
      frame "Events: Unregister" {
        # "Do not put any code in this frame.\n(It is a separator no-op. You can make a copy of this frame to create a new UI frame)"
        n117 = Unregister For Events(event registration refnum=w267, error in=w266) -> (error out=w265:errorcluster)
        n118 = call <vilib>:"Add State(s) to Queue__JKI_lib_State_Machine.vi"("State(s) in (\"\")"=w270) -> ("States Out"=w269:string)  [unwired: 14 in]
      }
      frame "---------- UI ----------" {
        # "Do not put any code in this frame.\n(It is a separator no-op. You can make a copy of this frame to create a new UI frame)"
        n119 = call <vilib>:"Add State(s) to Queue__JKI_lib_State_Machine.vi"("State(s) in (\"\")"=w275) -> ("States Out"=w274:string)  [unwired: 14 in]
      }
      frame "UI: Initialize" {
      }
      frame "UI: Cursor Set" {
        # "Argument"
        # "Set and Unset Cursor Busy.\n(Usage: \"UI: Cursor Set >> Busy|Idle\")"
        n120 = case shown="\"Idle\", Default" w281 {
          tunnel: w283 -> [w288 w290]
          tunnel: [w287 w289] -> w282
          frame "Idle", Default {
            n121 = call <vilib>:"Unset Busy.vi"("error in (no error)"=w288) -> ("error out"=w287:errorcluster)  [unwired: 10 in]
          }
          frame "Busy" {
            n122 = call <vilib>:"Set Busy.vi"("error in (no error)"=w290) -> ("error out"=w289:errorcluster)  [unwired: 9 in, 1 out]
          }
        }
        n123 = call <vilib>:"Add State(s) to Queue__JKI_lib_State_Machine.vi"("State(s) in (\"\")"=w286) -> ("States Out"=w285:string)  [unwired: 14 in]
      }
      frame "UI: Front Panel State" {
        # "Argument"
        # "Set Front Panel Open or Closed\n(Usage: \"UI: Front Panel State >> Open|Close\")"
        n124 = Unbundle By Name(w294) -> ("Core.Current VI Reference"=w293:refnum<vi>)
        n125 = case shown="\"Minimize\", \"Minimized\"" w292 {
          tunnel: w296 -> [w304 w319 w330 w343 w356]
          tunnel: [w306 w320 w332 w345 w358] -> w295
          tunnel: w293 -> [w305 w317 w331 w344 w357]
          frame "Open", "Standard", Default {
            w299 = T7."Standard" ("State")
            n126 = property class="VI"(reference=w305, error in=w304) -> (reference out=w302:refnum<vi>, error out=w303:errorcluster, "FP.State"=w301:T7)
            n127 = Not Equal?(x=w301, y=w299) -> (x != y?=w300:bool)
            n128 = case shown="True" w300 {
              tunnel: [w310 w312] -> w306
              tunnel: w303 -> [w309 w312]
              tunnel: w302 -> [w308 _]
              tunnel: w299 -> [w307 _]
              frame True {
                n129 = invoke class="VI" method="FP.Open"(reference=w308, error in=w309, "Activate"=TRUE, "State"=w307) -> (error out=w310:errorcluster)  [unwired: 1 in, 4 out]
              }
              frame False {
              }
            }
          }
          frame "Close", "Closed" {
            n130 = property class="VI"(reference=w317, error in=w319) -> (reference out=w316:refnum<vi>, error out=w318:errorcluster, "FP.State"=w314:T7)
            n131 = Not Equal?(x=w314, y=T7."Closed" ("Front Panel Window:State")) -> (x != y?=w313:bool)
            n132 = case shown="True" w313 {
              tunnel: [w321 w324] -> w320
              tunnel: w318 -> [w321 w323]
              tunnel: w316 -> [_ w322]
              frame False {
              }
              frame True {
                n133 = invoke class="VI" method="FP.Close"(reference=w322, error in=w323) -> (error out=w324:errorcluster)  [unwired: 1 in, 2 out]
              }
            }
          }
          frame "Hidden", "Hide" {
            w325 = T7."Hidden" ("State")
            n134 = property class="VI"(reference=w331, error in=w330) -> (reference out=w328:refnum<vi>, error out=w329:errorcluster, "FP.State"=w327:T7)
            n135 = Not Equal?(x=w327, y=w325) -> (x != y?=w326:bool)
            n136 = case shown="True" w326 {
              tunnel: [w336 w337] -> w332
              tunnel: w329 -> [w335 w337]
              tunnel: w328 -> [w334 _]
              tunnel: w325 -> [w333 _]
              frame True {
                n137 = invoke class="VI" method="FP.Open"(reference=w334, error in=w335, "State"=w333) -> (error out=w336:errorcluster)  [unwired: 2 in, 4 out]
              }
              frame False {
              }
            }
          }
          frame "Minimize", "Minimized" {
            w338 = T7."Minimized" ("State")
            n138 = property class="VI"(reference=w344, error in=w343) -> (reference out=w341:refnum<vi>, error out=w342:errorcluster, "FP.State"=w340:T7)
            n139 = Not Equal?(x=w340, y=w338) -> (x != y?=w339:bool)
            n140 = case shown="True" w339 {
              tunnel: [w349 w350] -> w345
              tunnel: w342 -> [w348 w350]
              tunnel: w341 -> [w347 _]
              tunnel: w338 -> [w346 _]
              frame True {
                n141 = invoke class="VI" method="FP.Open"(reference=w347, error in=w348, "State"=w346) -> (error out=w349:errorcluster)  [unwired: 2 in, 4 out]
              }
              frame False {
              }
            }
          }
          frame "Maximize", "Maximized" {
            w351 = T7."Maximized" ("State")
            n142 = property class="VI"(reference=w357, error in=w356) -> (reference out=w354:refnum<vi>, error out=w355:errorcluster, "FP.State"=w353:T7)
            n143 = Not Equal?(x=w353, y=w351) -> (x != y?=w352:bool)
            n144 = case shown="True" w352 {
              tunnel: [w362 w363] -> w358
              tunnel: w355 -> [w361 w363]
              tunnel: w354 -> [w360 _]
              tunnel: w351 -> [w359 _]
              frame True {
                n145 = invoke class="VI" method="FP.Open"(reference=w360, error in=w361, "State"=w359) -> (error out=w362:errorcluster)  [unwired: 2 in, 4 out]
              }
              frame False {
              }
            }
          }
        }
        n146 = call <vilib>:"Add State(s) to Queue__JKI_lib_State_Machine.vi"("State(s) in (\"\")"=w298) -> ("States Out"=w297:string)  [unwired: 14 in]
      }
      frame "---------- Macro ----------" {
        # "Do not put any code in this frame.\n(It is a separator no-op. You can make a copy of this frame to create a new Macro frame)"
        n147 = call <vilib>:"Add State(s) to Queue__JKI_lib_State_Machine.vi"("State(s) in (\"\")"=w368) -> ("States Out"=w367:string)  [unwired: 14 in]
      }
      frame "Macro: Initialize" {
        n148 = call <vilib>:"Add State(s) to Queue__JKI_lib_State_Machine.vi"("State(s) in Front (\"\")"="Data: Initialize\nInitialize Core Data\nEvents: Register\nUI: Initialize\n// UI: Front Panel State >> Open\n\n", "State(s) in (\"\")"=w374) -> ("States Out"=w373:string)  [unwired: 13 in]
      }
      frame "Macro: Update" {
        n149 = call <vilib>:"Add State(s) to Queue__JKI_lib_State_Machine.vi"("State(s) in Front (\"\")"="Action: Write Config", "State(s) in (\"\")"=w380) -> ("States Out"=w379:string)  [unwired: 13 in]
      }
      frame "Macro: Exit" {
        # "Exit Macro\n(This is called once, when the VI exits)"
        n150 = Unbundle By Name(w389) -> ("Core.Close Panel on Exit?"=w388:bool)
        n151 = Select(t="UI: Front Panel State >> Close", s=w388, f="") -> (s? t:f=w385:string)
        n152 = call <vilib>:"Add State(s) to Queue__JKI_lib_State_Machine.vi"("State(s) in Front (\"\")"="Action: Write Config", "State(s) in (\"\")"=w385, "State(s) at Back (\"\")"="Data: Cleanup\nEvents: Unregister\nExit") -> ("States Out"=w383:string)  [unwired: 12 in]
        n153 = call <vilib>:"Add State(s) to Queue__JKI_lib_State_Machine.vi"("State(s) in Front (\"\")"=w383, "State(s) in (\"\")"=w392) -> ("States Out"=w391:string)  [unwired: 13 in]
      }
      frame "---------- Action ----------" {
      }
      frame "Action: Write Config" {
        n154 = local read "Not Connect"() -> (w397:bool)
        n155 = case shown="False" w397 {
          tunnel: w401 -> [w408 w417]
          tunnel: [w410 w417] -> w400
          tunnel: w399 -> [w406 _]
          tunnel: w398 -> [w405 _]
          frame False {
            n156 = Unbundle By Name(w405) -> ("amc"=w413:refnum<class "MessageAMC.lvclass">)
            n157 = call "Read name.vi"("GUI in"=w406) -> ("name"=w407:string)  [unwired: 9 in, 1 out]
            n158 = call "Read SVW.vi"("GUI in"=w406) -> ("SharedVariableWrapper.lvclass"=w416:refnum<class "SharedVariableWrapper.lvclass">)  [unwired: 10 in]
            n159 = call "ReadConfig.vi"("SharedVariableWrapper in"=w416) -> ("config"=w415:T9)  [unwired: 12 in, 2 out]
            n160 = Unbundle By Name(w415) -> ("ip"=w414:string)
            n161 = call "SendNetworkVariant.vi"("reference in"=w413, "receiver process"=w407, "receiver host"=w414, "receiver port (0)"=u16 54321, "name"="SET_SETTINGS", "data"="Needle Valve Settings", "timeout (25000 ms)"=1000, "error in (no error)"=w408) -> ("error out"=w410:errorcluster)  [unwired: 5 in, 2 out]
          }
          frame True {
          }
        }
      }
    }
  }
  n162 = call "Read name.vi"("GUI in"=w4) -> ("name"=w7:string)  [unwired: 9 in, 1 out]
  n163 = call "Read SVW.vi"("GUI in"=w4) -> ("SharedVariableWrapper.lvclass"=w10:refnum<class "SharedVariableWrapper.lvclass">)  [unwired: 10 in]
  n164 = Concatenate Strings(w7, "_DATA" ("name")) -> (w6:string)
  n165 = property on="Engine State" class="Ring (strict)"() -> ("Strings []"=w9:string[])  [unwired: 2 in, 2 out]
  n166 = while {
    tunnel: w10 -> [w426]
    tunnel: w9 -> [w421]
    tunnel: w6 -> [w420]
    tunnel: w3 -> [w419]
    stop <- "stop" stop-if-true
    n167 = stacked-sequence {
      tunnel: w426 -> [w431 w454 w460]
      tunnel: [w447 _ _] -> w424
      tunnel: [_ w451 _] -> w425
      tunnel: w421 -> [w434 _ _]
      tunnel: w420 -> [w430 _ _]
      tunnel: w419 -> [_ _ w459]
      tunnel: [_ _ w458] -> w418
      frame #0 {
        n168 = call "Read.vim"("SharedVariableWrapper in"=w431, "name"=w430, "DataType"=T12 {"Engine State"=8, "StateValveModbus"=enum."STOPED", "Alarms"={"OL"=FALSE, "TF"=FALSE, "STL"=FALSE, "OCP"=FALSE, "CPUV"=FALSE, "UVLO"=FALSE, "SPI_ERROR"=FALSE, "Fault"=FALSE, "OL 2"=FALSE, "TF 2"=FALSE, "STL 2"=FALSE, "OCP 2"=FALSE, "CPUV 2"=FALSE, "UVLO 2"=FALSE, "reserved"=TRUE, "InitDone"=TRUE}, "RAW"=124110, "Angele"=0.0, "Step"=0, "Encoder"=0, "Kinematic"={"ACC Steps Per Sec^2"=100, "DEC Steps Per Sec^2"=100, "Min Velosity Step Per Sec"=100, "Max Velosity Step Per Sec"=200, "MicroStep"=16}, "Limits"={"Fault 2 Switch"=FALSE, "Fault 1 Switch"=FALSE, "Center(Home)"=FALSE, "Lower Limit"=FALSE, "Upper Limit"=FALSE}, "EncoderMax"=0, "Counter Max Dont Update"=0, "EncoderMin"=0, "Counter Min Dont Update"=0, "Prepere Counter"=0, "STEP INIT"=0, "offset - Angel"=0.0} ("NVM Data")) -> ("data out"=w445:T12, "error out"=w447:errorcluster)  [unwired: 6 in, 5 out]
        n169 = Unbundle By Name(w445) -> ("Limits"=→"Limits":T1, "Alarms"=→"Alarms":T6, "Engine State"=w433:T4, "StateValveModbus"=w435:T13, "offset - Angel"=→"Waveform Chart - Dark 3":dbl, "Step"=→"step":i32, "Encoder"=→"encoder":i32, "Kinematic"=→"Kinematic":T3)  [unwired: 6 out]
        n170 = Index Array(array=w434, index=w433) -> (element=w432:string)
        n171 = Format Into String(format string="VALVE STATE: %s ", w435) -> (resulting string=→"String 2":string)  [unwired: 2 in, 1 out]
        n172 = Format Into String(format string="DRIVER STATE: %s", w432) -> (resulting string=→"String":string)  [unwired: 2 in, 1 out]
      }
      frame #1 {
        n173 = call "Read.vim"("SharedVariableWrapper in"=w454, "name"="DO_ARRAY", "DataType"=bool[] []) -> ("data out"=w450:bool[], "error out"=w451:errorcluster)  [unwired: 6 in, 5 out]
        n174 = Index Array(array=w450, index=19) -> (element=→"DO 19":bool)
      }
      frame #2 {
        n175 = call "Read.vim"("SharedVariableWrapper in"=w460, "name"=w459, "DataType"=T2 {"average size"=0, "open force"=12, "close force"=12, "open settings"={"ACC Steps Per Sec^2"=0, "DEC Steps Per Sec^2"=0, "Min Velosity Step Per Sec"=0, "Max Velosity Step Per Sec"=0, "MicroStep"=0}, "close settings"={"ACC Steps Per Sec^2"=0, "DEC Steps Per Sec^2"=0, "Min Velosity Step Per Sec"=0, "Max Velosity Step Per Sec"=0, "MicroStep"=0}, "Offset angle"=0.0} ("Needle Valve Settings 2")) -> ("data out"=w456:T2, "error out"=w458:errorcluster)  [unwired: 6 in, 5 out]
        n176 = call "Is Value Changed.vim"("value"=w456) -> ("changed or first call?"=w455:bool)
        n177 = case shown="True" w455 {
          tunnel: w456 -> [_ w461]
          frame False {
          }
          frame True {
            n178 = local write "Needle Valve Settings"(w461) -> ()
          }
        }
      }
    }
    n179 = Merge Errors(w425, w424, w418) -> (w423:errorcluster)
    n180 = Wait Until Next ms Multiple(millisecond multiple=u32 100) -> ()  [unwired: 1 out]
    n181 = Unbundle By Name(w423) -> ("status"=→"Not Connect":bool)
  }
  n182 = flat-sequence {
    tunnel: w15 -> [w463]
    frame #0 {
      n183 = local write "stop"(TRUE ("stop")) -> ()
      "error out" <- w463
    }
  }
